vi "Increment.vi"(8 "error in (no error)":errorcluster, 10 "Numeric":dbl, 11 "TestActor in":refnum<class "Self Incrementer.lvclass">) -> (0 "error out":errorcluster, 3 "TestActor out":refnum<class "Self Incrementer.lvclass">)   [LabVIEW 2020, in "Messaging Tests.lvlib" / "Self Incrementer.lvclass"]
uses:
  Self Incrementer.lvclass
  C:/Users/J63553/Projects/_LabVIEW Community/actor-framework/Core/ActorFramework/Actor/Actor.lvclass
  Core/ActorFramework/Actor/Actor.lvclass/Actor.ctl
  Core/ActorFramework/Message Enqueuer/Message Enqueuer.lvclass/Message Enqueuer.ctl
  Self Incrementer.lvclass/Self Incrementer.ctl
  Start Increment Msg/Start Increment Msg.lvclass/Start Increment Msg.ctl
  Core/ActorFramework/Stop Msg/Stop Msg.lvclass/Stop Msg.ctl
  Core/ActorFramework/Message Enqueuer/Init from Existing Queue.vi
  Core/ActorFramework/Message Enqueuer/Enqueue.vi
  Core/ActorFramework/Message Enqueuer/Enqueue Critical.vi
  Start Increment Msg/Start Increment Msg.lvclass
  C:/Users/J63553/Projects/_LabVIEW Community/actor-framework/Core/ActorFramework/Message/Message.lvclass
  Core/ActorFramework/Stop Msg/Stop Msg.lvclass
  Core/ActorFramework/Message Priority Queue/Priority Enqueue.vi
  Core/ActorFramework/Message Enqueuer/Message Enqueuer.lvclass
  Core/ActorFramework/Actor/Actor.lvclass
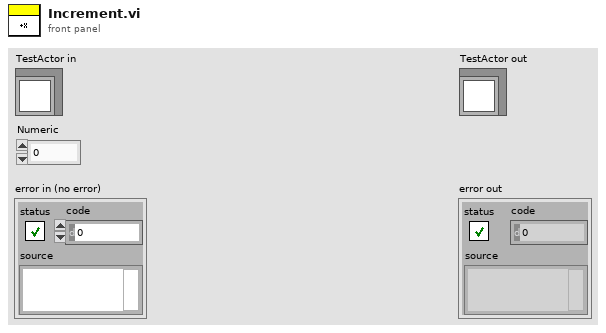
[diagram p1: front panel]
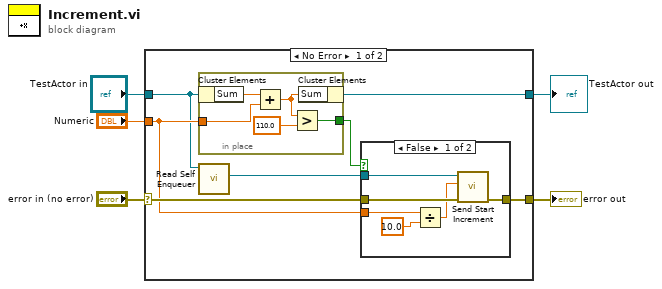
[diagram p0: block diagram]
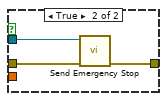
[diagram p2: hidden frame]
diagram:
  n1 = case shown="No Error" "error in (no error)" {
    selector: "error in (no error)" -> [w12 w28]
    tunnel: [w11 w28] -> w4
    tunnel: [w6 w27] -> w2
    tunnel: "TestActor in" -> [w8 w27]
    tunnel: "Numeric" -> [w9 _]
    frame No Error {
      n2 = in-place {
        in-place-border: w9 -> [w25]
        in-place-border: [w22] -> w10
        n3 = in-place-cluster #1(w8) -> ("Sum"=w26:dbl)
        n4 = Add(x=w26, y=w25) -> (x+y=w24:dbl)
        n5 = Greater?(x=w24, y=110.0) -> (0:w22:bool)
        n6 = in-place-cluster #1("Sum"=w24) -> (w6:refnum<class "Self Incrementer.lvclass">)
      }
      n7 = call "Read Self Enqueuer.vi"("Actor"=w8) -> ("Self Enqueuer"=w7:refnum<class "Message Enqueuer.lvclass">)  [unwired: 10 in]
      n8 = case shown="False" w10 {
        tunnel: w12 -> [w18 w21]
        tunnel: [w17 w20] -> w11
        tunnel: w7 -> [w16 w19]
        tunnel: w9 -> [w14 _]
        frame False {
          n9 = Divide(x=w14, y=10.0) -> (x/y=w13:dbl)
          n10 = call "Send Start Increment.vi"("error in (no error)"=w18, "Numeric"=w13, "Message Enqueuer"=w16) -> ("error out"=w17:errorcluster)  [unwired: 8 in]
        }
        frame True {
          n11 = call "Send Emergency Stop.vi"("error in (no error)"=w21, "Message Enqueuer"=w19) -> ("error out"=w20:errorcluster)  [unwired: 9 in]
        }
      }
    }
    frame Error {
    }
  }
  "error out" <- w4
  "TestActor out" <- w2
